vi "HFRR ADV v12.vi"() -> ()   [LabVIEW 2025] (continued)
    }
  }
  n4160 = stacked-sequence {
    tunnel: [w5562] -> w35
    frame #0 {
      w5562 = FALSE ("Upload \nConfirmed")
      n4161 = local write "Upload \nConfirmed"(w5562) -> ()
      n4162 = local write "St Str"("") -> ()
    }
  }
  n4163 = disable-structure shown="Disabled" {
    disable-tunnel: w35 -> [w5563 _]
    frame Disabled {
      n4164 = case shown="True" {
        selector: _ -> [_ _]
        tunnel: w5563 -> [_ w5564]
        frame False {
        }
        frame True {
          n4165 = while {
            tunnel: [w5570] -> _
            tunnel: w5564 -> [_]
            i -> [w5570]
            stop <- w5565 stop-if-true
            n4166 = local read "Json End Flg"() -> (w5569:bool)
            n4167 = Wait (ms)(milliseconds to wait=u32 20 ("Refresh Rate (ms)")) -> ()  [unwired: 1 out]
            n4168 = local read "refresh flag"() -> (w5566:bool)
            n4169 = local read "RUN"() -> (w5567:bool)
            n4170 = And(x=w5567, y=w5566) -> (x .and. y?=w5568:bool)
            n4171 = Or(x=w5568, y=w5569) -> (x .or. y?=w5571:bool)
            "AR Led" <- w5571
            n4172 = case shown="True" w5571 {
              frame False {
              }
              frame True {
                w5588 = "\",\""
                n4173 = local read "UUID"() -> (w5586:string)
                n4174 = local write "refresh flag"(FALSE ("refresh flag")) -> ()
                n4175 = local read "time"() -> (w5575:dbl)
                n4176 = Multiply(x=w5575, y=60.0) -> (x*y=w5574:dbl)
                n4177 = Concatenate Strings("UUID\" : \"", w5586, "\"}") -> (w5589:string)
                n4178 = Number To Fractional String(number=w5574, width (-)=i16 10, precision (6)=i16 4) -> (F-format string=w5603:string)  [unwired: 1 in]
                n4179 = Concatenate Strings("{", "\"Time\":\"", w5603, w5588) -> (w5598:string)
                n4180 = stacked-sequence {
                  tunnel: w5588 -> [w5651 w5659 w5666 w5674 w5682 w5691 w5698]
                  tunnel: [w5652 _ _ _ _ _ _] -> w5602
                  tunnel: [_ w5660 _ _ _ _ _] -> w5601
                  tunnel: [_ _ w5667 _ _ _ _] -> w5600
                  tunnel: [_ _ _ w5676 _ _ _] -> w5599
                  tunnel: w5589 -> [_ _ _ _ _ _ w5709]
                  tunnel: [_ _ _ _ _ _ w5708] -> w5585
                  tunnel: [_ _ _ _ _ w5688 _] -> w5584
                  tunnel: [_ _ _ _ w5681 _ _] -> w5583
                  frame #0 {
                    n4181 = local read "NORMAL LOAD"() -> (w5650:dbl)
                    n4182 = Number To Fractional String(number=w5650, width (-)=i16 10, precision (6)=i16 4) -> (F-format string=w5653:string)  [unwired: 1 in]
                    n4183 = Concatenate Strings("NormalLoad\":\"", w5653, w5651) -> (w5652:string)
                  }
                  frame #1 {
                    n4184 = local read "Temp"() -> (w5658:dbl)
                    n4185 = Number To Fractional String(number=w5658, width (-)=i16 10, precision (6)=i16 4) -> (F-format string=w5661:string)  [unwired: 1 in]
                    n4186 = Concatenate Strings("Temperature\":\"", w5661, w5659) -> (w5660:string)
                  }
                  frame #2 {
                    n4187 = local read "cof"() -> (w5664:dbl)
                    n4188 = Number To Fractional String(number=w5664, width (-)=i16 10, precision (6)=i16 4) -> (F-format string=w5668:string)  [unwired: 1 in]
                    n4189 = Concatenate Strings("FrictionalForce\":\"", w5668, w5666) -> (w5667:string)
                  }
                  frame #3 {
                    n4190 = local read "Set Hz"() -> (w5672:dbl)
                    n4191 = Multiply(x=w5672, y=60.0) -> (x*y=w5671:dbl)
                    n4192 = Number To Fractional String(number=w5671, width (-)=i16 10, precision (6)=i16 4) -> (F-format string=w5677:string)  [unwired: 1 in]
                    n4193 = Concatenate Strings("Speed\":\"", w5677, w5674) -> (w5676:string)
                  }
                  frame #4 {
                    n4194 = local read "Stroke Ln"() -> (w5680:dbl)
                    n4195 = Number To Fractional String(number=w5680, width (-)=i16 10, precision (6)=i16 4) -> (F-format string=w5684:string)  [unwired: 1 in]
                    n4196 = Concatenate Strings("LinearDeformation\":\"", w5684, w5682) -> (w5681:string)
                  }
                  frame #5 {
                    n4197 = local read "AIR TEMP"() -> (w5687:dbl)
                    n4198 = local read "Json St Flg"() -> (w5689:bool)
                    n4199 = local read "Json End Flg"() -> (w5690:bool)
                    n4200 = Number To Fractional String(number=w5687, width (-)=i16 10, precision (6)=i16 4) -> (F-format string=w5693:string)  [unwired: 1 in]
                    n4201 = Concatenate Strings("Vibration\":\"", w5693, w5691) -> (w5688:string)
                    n4202 = And(x=w5689, y=w5690) -> ()  [unwired: 1 out]
                  }
                  frame #6 {
                    n4203 = local read "Json End Flg"() -> (w5697:bool)
                    n4204 = Get Date/Time In Seconds() -> (seconds since 1Jan1904=w5705:timestamp)
                    n4205 = local read "Json St Flg"() -> (w5696:bool)
                    n4206 = To Double Precision Float(number=w5705) -> (double precision float=w5704:dbl)
                    n4207 = Subtract(x=w5704, y=2082844800.0) -> (x-y=w5702:dbl)
                    n4208 = Number To Fractional String(number=w5702, width (-)=i16 12, precision (6)=i16 0) -> (F-format string=w5699:string)  [unwired: 1 in]
                    n4209 = case shown="True" w5697 {
                      tunnel: ["" w5712] -> w5706
                      tunnel: w5699 -> [_ w5713]
                      tunnel: w5698 -> [_ w5711]
                      frame False {
                      }
                      frame True {
                        n4210 = local write "Json End Flg"(FALSE ("Json St Flg")) -> ()
                        n4211 = Concatenate Strings("End\": \"", w5713, w5711) -> (w5712:string)
                      }
                    }
                    n4212 = case shown="True" w5696 {
                      tunnel: [w5716 w5719] -> w5707
                      tunnel: w5699 -> [_ w5720]
                      tunnel: w5698 -> [_ w5717]
                      frame False {
                        n4213 = local read "St Str"() -> (w5716:string)
                      }
                      frame True {
                        n4214 = Concatenate Strings("Start\":\"", w5720, w5717) -> (w5719:string)
                        "St Str" <- w5719
                        n4215 = local write "Json St Flg"(FALSE ("Json St Flg")) -> ()
                      }
                    }
                    n4216 = Concatenate Strings(w5707, w5706, w5709) -> (w5708:string)
                  }
                }
                n4217 = local read "FILE"() -> (w5577:string)
                n4218 = Concatenate Strings("\",\"OperatorID\":\"" ("string"), "Operator ID") -> (w5580:string)
                n4219 = Concatenate Strings("\",\"DatasetTitle\":\"" ("string"), w5577) -> (w5579:string)
                n4220 = Concatenate Strings("\",\"SerialNumber\":\"" ("string"), "Serial No") -> (w5609:string)
                n4221 = Concatenate Strings("\",\"ModelNumber\":\"" ("string"), "Model No") -> (w5608:string)
                n4222 = Concatenate Strings(w5609, w5608) -> (w5591:string)
                n4223 = Concatenate Strings("{\"SecretKey\":\"", "Secret Key", w5591, w5580, w5579, "\",\"Samples\":[") -> (w5596:string)
                n4224 = Concatenate Strings(w5598, w5602, w5601, w5600, w5599, w5583, w5584, w5585) -> (w5597:string)
                n4225 = Concatenate Strings(w5596, w5597, "]}") -> (w5595:string)
                n4226 = stacked-sequence {
                  tunnel: w5595 -> [w5624 _ _]
                  tunnel: [_ _ w5641] -> _
                  frame #0 {
                    (unwired) FALSE ("convert eol (F)")
                    w5626 = enum16{"start", "end", "current"}."start" ("pos mode (0:2)")
                    n4227 = Path To String(path="Path") -> (string=w5632:string)
                    n4228 = Concatenate Strings(w5632, "\\", "Data File Name") -> (w5634:string)
                    n4229 = local write "standard output"(" ") -> ()
                    n4230 = String To Path(string=w5634) -> (path=w5623:path)
                    n4231 = call <vilib>:"Open_Create_Replace File.vi"("advisory dialog? (display:T)"=FALSE, "function (open:0)"=T28."create or replace", "file path"=w5623) -> ("error out"=w5637:errorcluster, "refnum"=w5636:refnum<file>)  [unwired: 5 in, 2 out]
                    n4232 = Set File Position(refnum=w5636, from (0:start)=w5626, error in=w5637) -> (refnum out=w5617:refnum<file>, error out=w5616:errorcluster)  [unwired: 1 in]
                    n4233 = Write to Binary File(file (use dialog)=w5617, data=" ", error in=w5616, 5:FALSE ("prepend array or string size? (T)")) -> (refnum out=w5627:refnum<file>, error out=w5628:errorcluster)  [unwired: 2 in, 1 out]
                    n4234 = Set File Position(offset (in bytes) (0)=w5626, refnum=w5627, error in=w5628) -> (refnum out=w5620:refnum<file>, error out=w5619:errorcluster)  [unwired: 1 in]
                    n4235 = Write to Binary File(file (use dialog)=w5620, data=w5624, error in=w5619, 5:FALSE ("prepend array or string size? (T)")) -> (error out=w5622:errorcluster)  [unwired: 2 in, 2 out]
                    n4236 = flat-sequence {
                      tunnel: w5623 -> [w5639]
                      tunnel: w5622 -> [_]
                      frame #0 {
                        n4237 = call <vilib>:"Read Characters From File.vi"("file path (dialog if empty)"=w5639) -> ("character string"=→"JSON string":string)  [unwired: 5 in, 3 out]
                      }
                    }
                    "SinglePoint" <- w5624
                  }
                  frame #1 {
                  }
                  frame #2 {
                    (unwired) "\"Stored\": true" ("string")
                    n4238 = call <vilib>:"System Exec.vi"("run minimized? (F)"=TRUE, "wait until completion? (T)"=TRUE, "working directory"=path "C:/LAB-IQ-NXT", "command line"="C:\\LAB-IQ-NXT\\JPost.bat") -> ("standard error"=→"Respose From Server":string, "standard output"=w5644:string)  [unwired: 4 in, 2 out]
                    "standard output" <- w5644
                    n4239 = Match Pattern(string=w5644, regular expression="JSON Check String") -> (match substring=w5642:string, offset past match=w5641:i32)  [unwired: 1 in, 2 out]
                    n4240 = Equal?(x=w5642, y="JSON Check String") -> (x = y?=→"Upload \nConfirmed":bool)
                  }
                }
              }
            }
            n4241 = local read "Quit"() -> (w5565:bool)
          }
        }
      }
    }
    frame Enabled {
    }
  }
  n4242 = disable-structure shown="Disabled" {
    disable-tunnel: _ -> [w5727 _]
    frame Disabled {
      n4243 = while {
        shift-right: [w5735] -> w5723
        shift-left: _ -> [w5736]
        shift-right: [w5733] -> w5724
        shift-left: errorcluster {"status"=TRUE, "code"=0, "source"="Init"} ("error out") -> [w5734]
        shift-right: [w5731] -> _
        shift-left: "" -> [w5732]
        tunnel: [w5729] -> _
        tunnel: w5727 -> [_]
        i -> [w5729]
        stop <- w5728 stop-if-true
        n4244 = flat-sequence {
          tunnel: [w5737] -> w5730
          frame #0 {
            n4245 = Wait (ms)(milliseconds to wait=10.0 ("Delay")) -> (millisecond timer value=w5737:u32)
          }
        }
        n4246 = case shown="No Error" w5734 {
          selector: w5734 -> [w5770 w5892]
          tunnel: [w5752 w5894] -> w5735
          tunnel: [w5751 w5893] -> w5733
          tunnel: w5736 -> [w5771 w5886]
          tunnel: w5732 -> [w5750 w5885]
          tunnel: [w5749 w5885] -> w5731
          tunnel: w5730 -> [_ _]
          frame No Error {
            n4247 = Concatenate Strings("COMMAND", "\r", "\n") -> (w5761:string)
            n4248 = case shown="True" "Measure" {
              tunnel: w5771 -> [w5797 w5804]
              tunnel: w5770 -> [w5796 w5803]
              tunnel: [w5797 w5802] -> w5769
              tunnel: [w5796 w5801] -> w5748
              tunnel: w5761 -> [_ w5800]
              frame False {
              }
              frame True {
                n4249 = VISA Write(VISA resource name=w5804, write buffer=w5800, error in (no error)=w5803) -> (VISA resource name out=w5802:refnum<visa-resource-name>, error out=w5801:errorcluster)  [unwired: 1 out]
                n4250 = local write "Read String"("") -> ()
                n4251 = local write "Measure"(FALSE) -> ()
              }
            }
            n4252 = property class="Instr"(reference=w5769, error in=w5748) -> (reference out=w5768:refnum<visa-resource-name>, error out=w5767:errorcluster, "Serial Settings:Number of Bytes at Serial Port"=w5766:u32)
            n4253 = Greater?(x=w5766, y=u32 100) -> (0:w5764:bool)
            n4254 = case shown="True" w5764 {
              tunnel: w5768 -> [w5807 w5832]
              tunnel: w5767 -> [w5806 w5831]
              tunnel: w5766 -> [_ w5830]
              tunnel: [w5807 w5829] -> w5754
              tunnel: [w5806 w5828] -> w5753
              tunnel: w5750 -> [w5805 w5827]
              tunnel: [w5805 ""] -> w5749
              frame False {
              }
              frame True {
                w5817 = u32 6 ("y")
                # "Page 84 of \nmanual"
                n4255 = VISA Read(VISA resource name=w5832, byte count=w5830, error in (no error)=w5831) -> (VISA resource name out=w5829:refnum<visa-resource-name>, read buffer=w5825:string, error out=w5828:errorcluster)  [unwired: 1 out]
                n4256 = while {
                  tunnel: w5825 -> [w5881]
                  tunnel: [w5877] -> w5819 mode=indexing
                  tunnel: [w5871] -> w5823 mode=indexing
                  tunnel: [w5869] -> _
                  i -> [w5869]
                  stop <- w5874 stop-if-true
                  n4257 = String Subset(string=w5881, offset (0)=w5869) -> (substring=w5876:string)  [unwired: 1 in]
                  n4258 = String To Byte Array(string=w5876) -> (unsigned byte array=w5880:u8[])
                  n4259 = String Length(string=w5876) -> (length=w5875:i32)
                  n4260 = Index Array(array=w5880) -> (element=w5879:u8)  [unwired: 1 in]
                  n4261 = Equal To 0?(x=w5875) -> (x = 0?=w5874:bool)
                  n4262 = Number To Boolean Array(number=w5879) -> (Boolean array=w5873:bool[])
                  n4263 = Reverse 1D Array(array=w5873) -> (reversed array=w5872:bool[])
                  n4264 = And(x=w5873, y=bool[] [FALSE, FALSE, FALSE, FALSE, FALSE, FALSE, TRUE, TRUE] ("Boolean array")) -> (x .and. y?=w5877:bool[])
                  n4265 = And(x=w5872, y=bool[] [FALSE, FALSE, TRUE, TRUE, TRUE, TRUE, TRUE, TRUE] ("Boolean array")) -> (x .and. y?=w5871:bool[])
                }
                n4266 = Concatenate Strings(w5827, w5825) -> (→"Read String":string)
                n4267 = while {
                  tunnel: w5819 -> [w5868] mode=indexing
                  tunnel: [w5864] -> w5822
                  i -> [w5864]
                  stop <- w5865 stop-if-true
                  n4268 = Search 1D Array(1D array=w5868, element=TRUE) -> (index of element=w5866:i32)  [unwired: 1 in]
                  n4269 = Less Than 0?(x=w5866) -> (x < 0?=w5865:bool)
                }
                n4270 = Delete From Array(array=w5823, length=w5822, index (row)=0) -> (array with subset deleted=w5818:bool[][])  [unwired: 1 in, 1 out]
                n4271 = Array Size(array=w5818) -> (size(s)=w5820:i32[])
                n4272 = Index Array(array=w5820) -> (element=w5812:i32)  [unwired: 1 in]
                n4273 = Greater?(x=w5812, y=w5817) -> (0:w5815:bool)
                n4274 = Subtract(x=w5812, y=w5817) -> (x-y=w5816:u32)
                n4275 = Select(t=w5816, s=w5815, f=u32 0) -> (s? t:f=w5813:u32)
                n4276 = while {
                  tunnel: w5818 -> [w5851]
                  tunnel: [w5853] -> w5811 mode=indexing
                  tunnel: w5813 -> [w5835]
                  i -> [w5852]
                  stop <- w5850 stop-if-true
                  w5842 = 6 ("index")
                  w5841 = 2 ("length")
                  # "Page 65 of \nmanual"
                  n4277 = Multiply(x=u32 3 ("y"), y=w5852) -> (x*y=w5849:u32)
                  n4278 = Divide(x=u32 102 ("y"), y=u32 65520) -> (x/y=w5859:dbl)
                  n4279 = Greater Or Equal?(x=w5849, y=w5835) -> (x >= y?=w5850:bool)
                  n4280 = Index Array(array=w5851, index (row) #1=w5849) -> (element #1=w5847:bool[], element #2=w5846:bool[], element #3=w5845:bool[])  [unwired: 5 in]
                  n4281 = Reverse 1D Array(array=w5847) -> (reversed array=w5840:bool[])
                  n4282 = Reverse 1D Array(array=w5846) -> (reversed array=w5844:bool[])
                  n4283 = Reverse 1D Array(array=w5845) -> (reversed array=w5843:bool[])
                  n4284 = Delete From Array(array=w5840, length=w5841, index=w5842) -> (array with subset deleted=w5836:bool[])  [unwired: 1 out]
                  n4285 = Delete From Array(array=w5844, length=w5841, index=w5842) -> (array with subset deleted=w5837:bool[])  [unwired: 1 out]
                  n4286 = Delete From Array(array=w5843, length=w5841, index=w5842) -> (array with subset deleted=w5838:bool[])  [unwired: 1 out]
                  n4287 = Insert Into Array(array=bool[] [] ("Boolean array"), new element #1=w5836, new element #2=w5837, new element #3=w5838) -> (w5839:bool[])  [unwired: 1 in]
                  n4288 = Boolean Array To Number(Boolean array=w5839) -> (number=w5848:u32)
                  n4289 = Multiply(x=w5859, y=w5848) -> (x*y=w5858:dbl)
                  n4290 = Decrement(x=w5858) -> (x-1=w5857:dbl)
                  n4291 = Divide(x=w5857, y=u32 100) -> (x/y=w5855:dbl)
                  n4292 = Multiply(x=w5855, y=u32 10) -> (x*y=w5853:dbl)
                }
                n4293 = Delete From Array(array=w5811) -> (array with subset deleted=w5810:dbl[])  [unwired: 2 in, 1 out]
                "Waveform Graph 5" <- w5810
                "Waveform Chart 3" <- w5810
                n4294 = call-poly <vilib>:"Mean.vi"("X"=w5810) -> ("mean"=w5809:dbl)  [unwired: 1 out]
                "Measure_LDS" <- w5809
                n4295 = case shown="True" "Zero 4" {
                  tunnel: w5809 -> [_ w5834]
                  frame False {
                  }
                  frame True {
                    n4296 = local write "Zero 4"(FALSE ("Zero 4")) -> ()
                    "z_measure" <- w5834
                  }
                }
              }
            }
            n4297 = local read "Measure_LDS"() -> (w5744:dbl)
            n4298 = local read "Disp (mm)"() -> (w5743:dbl)
            n4299 = local read "Boolean 7"() -> (w5742:bool)
            n4300 = local read "Boolean 8"() -> (w5741:bool)
            n4301 = case shown="True" "Boolean 8" {
              tunnel: w5743 -> [_ w5774]
              tunnel: w5744 -> [_ w5773]
              frame False {
              }
              frame True {
                n4302 = local read "Captured Values 2"() -> (w5777:dbl[][])
                n4303 = Build Array(w5774, w5773) -> (w5772:dbl[])
                n4304 = Build Array (concatenate)(w5777, w5772) -> (w5775:dbl[][])
                n4305 = local write "Captured Values 2"(w5775) -> ()
                n4306 = local write "Boolean 8"(FALSE ("Boolean 8")) -> ()
              }
            }
            n4307 = call "Build XY Graph"("Enable"=w5741, "Reset"=w5742, "Y Input"=w5744, "X Input"=w5743) -> ("XY Graph"=→"?":cluster{"Y":dbl[], "Y":dbl[]}[])  [unwired: 6 in, 1 out]
            n4308 = case shown="True" "Boolean 9" {
              frame False {
              }
              frame True {
                n4309 = local read "Captured Values 2"() -> (w5779:dbl[][])
                n4310 = Index Array(array=w5779, index (col) #1=0 ("disabled index (col)"), index (col) #2=1 ("index (col)")) -> (element #1=w5782:dbl[], element #2=w5781:dbl[])  [unwired: 2 in]
                n4311 = call <vilib>:"Linear Fit.vi"("Y"=w5782, "X"=w5781) -> ("slope"=→"Slope":dbl, "intercept"=→"Intercept":dbl)  [unwired: 9 in, 3 out]
                n4312 = local write "Boolean 9"(FALSE ("Boolean 9")) -> ()
              }
            }
            n4313 = case shown="True" "Boolean 7" {
              frame False {
              }
              frame True {
                n4314 = local write "Captured Values 2"(dbl[][] [] ("Captured Values")) -> ()
                n4315 = local write "Boolean 7"(FALSE ("Boolean 7")) -> ()
              }
            }
            n4316 = Concatenate Strings("COMMAND 2", "\r", "\n") -> (w5756:string)
            n4317 = case shown="True" "Measure 2" {
              tunnel: w5754 -> [w5789 w5795]
              tunnel: w5753 -> [w5788 w5794]
              tunnel: [w5789 w5793] -> w5752
              tunnel: [w5788 w5792] -> w5751
              tunnel: w5756 -> [_ w5791]
              frame False {
              }
              frame True {
                n4318 = local write "Measure 2"(FALSE ("WRITE")) -> ()
                n4319 = VISA Write(VISA resource name=w5795, write buffer=w5791, error in (no error)=w5794) -> (VISA resource name out=w5793:refnum<visa-resource-name>, error out=w5792:errorcluster)  [unwired: 1 out]
              }
            }
          }
          frame Error {
            w5884 = u16 10 items=["1.0"=10, "1.5"=15, "2.0"=20] ("stop bits (10: 1 bit)")
            n4320 = Wait (ms)(milliseconds to wait=u32 20) -> ()  [unwired: 1 out]
            n4321 = VISA Close(VISA resource name=w5886, error in (no error)=w5892) -> (error out=w5891:errorcluster)
            n4322 = call <vilib>:"Clear Errors.vi"("error in (no error)"=w5891) -> ("error out"=w5890:errorcluster)  [unwired: 5 in, 1 out]
            n4323 = call-poly "VISA Configure Serial Port"("VISA resource name"="Laser Disp Sensor", "timeout (10sec)"=u32 200, "Enable Termination\nChar (T)"=TRUE ("Enable Termination\nChar (T)"), "baud rate (9600)"=u32 921600, "error in (no error)"=w5890, "stop bits (10: 1 bit)"=w5884) -> ("VISA resource name out"=w5894:refnum<visa-resource-name>, "error out"=w5893:errorcluster)  [unwired: 8 in]
          }
        }
        n4324 = local read "Quit"() -> (w5728:bool)
      }
      n4325 = VISA Close(VISA resource name=w5723, error in (no error)=w5724) -> (error out=w5722:errorcluster)
      n4326 = call <vilib>:"Clear Errors.vi"("error in (no error)"=w5722) -> ()  [unwired: 5 in, 2 out]
    }
    frame Enabled {
    }
  }
  n4327 = disable-structure shown="Disabled" {
    disable-tunnel: _ -> [w5899 _]
    frame Disabled {
      n4328 = while {
        tunnel: [w5906] -> _
        shift-right: [w5903] -> w5896
        shift-left: _ -> [w5905]
        shift-right: [w5904] -> w5897
        shift-left: errorcluster {"status"=TRUE, "code"=0, "source"="Init"} ("error out") -> [w5902]
        tunnel: w5899 -> [_]
        i -> [w5906]
        stop <- w5900 stop-if-true
        n4329 = flat-sequence {
          tunnel: w5902 -> [w5997]
          tunnel: [w5997] -> w5901
          frame #0 {
            n4330 = Wait (ms)(milliseconds to wait=u32 50) -> ()  [unwired: 1 out]
          }
        }
        n4331 = case shown="No Error" w5901 {
          selector: w5901 -> [w5947 w5990]
          tunnel: w5905 -> [w5946 w5989]
          tunnel: [w5913 w5980] -> w5904
          tunnel: [w5914 w5988] -> w5903
          frame No Error {
            w5940 = T29 {"Mode"=enum."RTU", "Slave Address"=1} ("Serial Parameters")
            n4332 = call-poly <vilib>:"MB Serial Master Query (poly).vi"("VISA resource name"=w5946, "Starting Address"=i16 1000, "Quantity"=u16 1, "Timeout"=u32 1000, "error in"=w5947, "Serial Parameters"=w5940) -> ("VISA resource name out"=w5941:refnum<visa-resource-name>, "Input Registers"=w5943:u16[], "error out"=w5939:errorcluster)  [unwired: 10 in, 1 out]
            n4333 = Random Number (0-1)() -> (number: 0 to 1=w5928:dbl)
            n4334 = Index Array(array=w5943, index=0) -> (element=w5938:u16)
            n4335 = Subtract(x=w5928, y=0.5) -> (x-y=w5927:dbl)
            n4336 = Divide(x=w5938, y=10 ("index")) -> (x/y=w5932:dbl)
            n4337 = Multiply(x=w5927, y=0.5) -> (x*y=w5926:dbl)
            n4338 = Add(x=w5932, y=w5926) -> (x+y=w5931:dbl)
            n4339 = local read "Amb temp"() -> (w5915:dbl)
            n4340 = Multiply(x=w5931, y=0.2) -> (x*y=w5935:dbl)
            n4341 = Multiply(x=w5915, y=0.8) -> (x*y=w5933:dbl)
            n4342 = Add(x=w5935, y=w5933) -> (x+y=w5916:dbl)
            n4343 = local read "set temp old"() -> (w5910:dbl)
            n4344 = local write "Amb temp"(w5916) -> ()
            n4345 = Select(t="SetTemp 2", s="Heater", f=100.0) -> (s? t:f=w5911:dbl)
            n4346 = Not Equal?(x=w5911, y=w5910) -> (x != y?=w5909:bool)
            n4347 = case shown="True" w5909 {
              tunnel: w5941 -> [w5975 w5977]
              tunnel: [w5974 w5977] -> w5921
              tunnel: w5939 -> [w5973 w5976]
              tunnel: [w5972 w5976] -> w5919
              tunnel: w5911 -> [w5967 _]
              tunnel: w5940 -> [w5969 w5978]
              tunnel: [w5969 w5978] -> w5922
              frame True {
                n4348 = Multiply(x=w5967, y=10 ("index")) -> (x*y=w5966:dbl)
                n4349 = call-poly <vilib>:"MB Serial Master Query (poly).vi"("VISA resource name"=w5975, "Address"=u16 0, "Holding Register"=w5966, "Timeout"=u32 1000, "error in"=w5973, "Serial Parameters"=w5969) -> ("VISA resource name out"=w5974:refnum<visa-resource-name>, "error out"=w5972:errorcluster)  [unwired: 11 in, 1 out]
                "set temp old" <- w5967
              }
              frame False {
              }
            }
            n4350 = flat-sequence {
              tunnel: [w5948] -> _
              tunnel: [w5948] -> w5918
              tunnel: w5919 -> [w5948]
              frame #0 {
                n4351 = Wait (ms)(milliseconds to wait=u32 100) -> ()  [unwired: 1 out]
              }
            }
            n4352 = call "Elapsed Time12"("Time Target (s)"=2.0, "Auto Reset"=TRUE) -> ("Time has Elapsed"=w5923:bool)  [unwired: 10 in, 7 out]
            n4353 = case shown="True" w5923 {
              tunnel: w5922 -> [w5952 w5965]
              tunnel: [w5952 w5965] -> _
              tunnel: [w5951 w5963] -> w5914
              tunnel: w5921 -> [w5951 w5964]
              tunnel: [w5950 w5961] -> w5913
              tunnel: w5918 -> [w5950 w5962]
              frame False {
              }
              frame True {
                n4354 = call-poly <vilib>:"MB Serial Master Query (poly).vi"("VISA resource name"=w5964, "Starting Address"=i16 1003 ("Addr"), "Quantity"=u16 1, "Timeout"=u32 1000, "error in"=w5962, "Serial Parameters"=w5965) -> ("VISA resource name out"=w5963:refnum<visa-resource-name>, "Input Registers"=w5958:u16[], "error out"=w5961:errorcluster)  [unwired: 10 in, 1 out]
                n4355 = Index Array(array=w5958, index=0) -> (element=w5957:u16)
                n4356 = Divide(x=w5957, y=u16 10) -> (x/y=w5953:dbl)
                n4357 = local write "set temp old"(w5953) -> ()
                n4358 = local write "SetTemp"(w5953) -> ()
              }
            }
            "Error Code" <- w5913
            n4359 = Unbundle(w5913) -> ("status"=→"TK4 status":bool)  [unwired: 2 out]
            "SetTemp" <- "SetTemp 2"
          }
          frame Error {
            w5992 = u16 0 items=["None", "Odd", "Even", "Mark", "Space"] ("Parity")
            w5993 = u16 0 items=["None", "XON/XOFF", "RTS/CTS", "XON/XOFF & RTS/CTS", "DTR/DSR", "XON/XOFF & DTR/DSR"] ("Flow Control")
            n4360 = VISA Clear(VISA resource name=w5989, error in (no error)=w5990) -> (VISA resource name out=w5983:refnum<visa-resource-name>, error out=w5981:errorcluster)
            n4361 = VISA Close(VISA resource name=w5983, error in (no error)=w5981) -> (error out=w5982:errorcluster)
            n4362 = call <vilib>:"Clear Errors.vi"("error in (no error)"=w5982) -> ("error out"=w5991:errorcluster)  [unwired: 5 in, 1 out]
            n4363 = Unbundle By Name(T29 {"Mode"=enum."RTU", "Slave Address"=1} ("input cluster")) -> ("Mode"=w5994:enum16{"RTU", "ASCII"})
            n4364 = call <vilib>:"MB Serial Init.vi"("Timeout"=u32 100, "Flow Control"=w5993, "Mode"=w5994, "error in (no error)"=w5991, "Parity"=w5992, "Baud Rate"=u32 9600, "VISA resource name"="Lubrication System COM Port :") -> ("error out"=w5980:errorcluster, "VISA resource name out"=w5988:refnum<visa-resource-name>)  [unwired: 3 in]
            n4365 = local write "set temp old"(0.0 ("set temp old")) -> ()
            n4366 = Unbundle(w5980) -> ("status"=w5979:bool)  [unwired: 2 out]
            n4367 = case shown="True" w5979 {
              selector: w5979 -> [_ w5996]
              frame False {
              }
              frame True {
                n4368 = local write "TK4 status"(w5996) -> ()
              }
            }
          }
        }
        n4369 = local read "Quit"() -> (w5900:bool)
      }
      n4370 = VISA Close(VISA resource name=w5896, error in (no error)=w5897) -> (error out=w5895:errorcluster)
      n4371 = call <vilib>:"Clear Errors.vi"("error in (no error)"=w5895) -> ()  [unwired: 5 in, 2 out]
    }
    frame Enabled {
    }
  }
  "file count" <- 0 ("file count")
